vi "Variable globale.vi"() -> ()   [LabVIEW 2017]
panel:
  out "x- last state":bool
  out "x+ last state":bool
  in  "Speed":dbl
  out "z+y- last state":bool
  out "z-y+ last state":bool
  out "z-y- last state":bool
  out "z+y+ last state":bool
  out "y- last state":bool
  out "y+ last state":bool
  out "z- last state":bool
  out "z+ last state":bool
  out "- last state":bool
  out "+ last state":bool
  in  "Ressolution Codeur":dbl
  in  "Pulse/Degre":dbl
  in  "Diametre Galet Codeur":dbl
  in  "Diametre Plateau":dbl
  in  "Decel Max":dbl
  in  "Accel Max":dbl
  in  "VMax":dbl
  in  "Decel":dbl
  in  "Accel":dbl
  # "Param Utilisateur"
  # "Param Système"
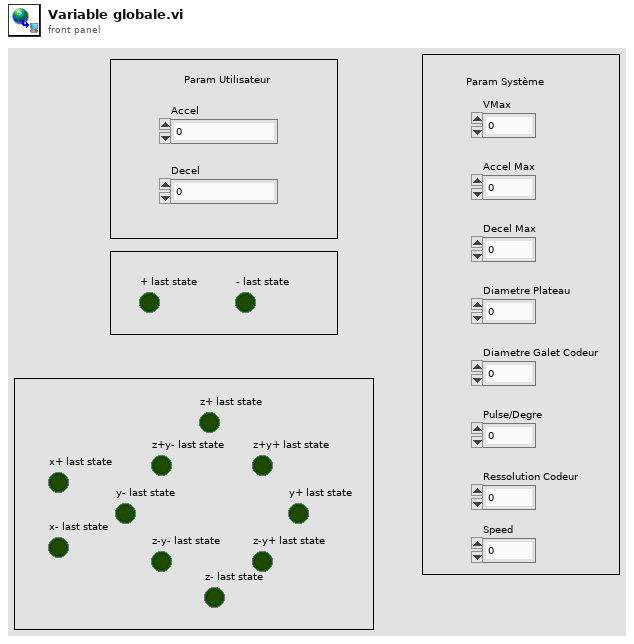
[diagram p1: front panel]
diagram:
